vi "WPI_DigitalModuleERRDIOAlreadyAllocated.vi"(8 "error in (no error)":errorcluster, 10 "DIOChannel":T1) -> (0 "error out":errorcluster)   [LabVIEW 2017]
doc: "This software is licensed. Open the labview\\readme\\WPI Robotics Library Open Source License.txt file for more information."
uses:
  <vilib>/Rock Robotics/SystemInterfaces/DIO/FPGA_DIOChannel.ctl
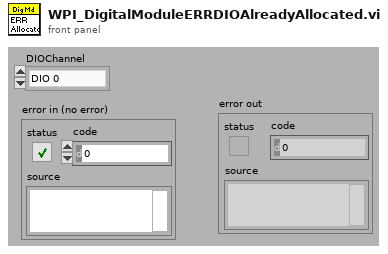
[diagram p1: front panel]
types:
  T1 = typedef "FPGA_DIOChannel.ctl" = enum8{"DIO 0", "DIO 1", "DIO 2", "DIO 3", "DIO 4", "DIO 5", "DIO 6", "DIO 7", "DIO 8", "DIO 9", "DIO MXP 0", "DIO MXP 1", "DIO MXP 2", "DIO MXP 3", "DIO MXP 4", "DIO MXP 5", "DIO MXP 6", "DIO MXP 7", "DIO MXP 8", "DIO MXP 9", "DIO MXP 10", "DIO MXP 11", "DIO MXP 12", "DIO MXP 13", "DIO MXP 14", "DIO MXP 15", "SPI Port CS1", "SPI Port CS2", "SPI Port CS3", "SPI Port MISO", "SPI Port MOSI", "Invalid"}
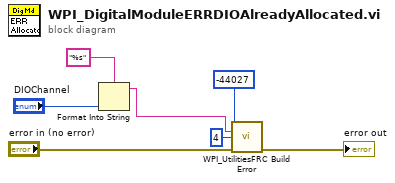
[diagram p0: block diagram]
diagram:
  n1 = Format Into String(format string="%s", "DIOChannel") -> (resulting string=w2:string)  [unwired: 2 in, 1 out]
  n2 = call <vilib>:"WPI_UtilitiesFRC Build Error.vi"("error code"=-44027 ("code"), "extra error text"=w2, "chain levels to remove (1)"=4, "error in (no error)"="error in (no error)") -> ("error out"=→"error out":errorcluster)  [unwired: 1 in, 10 out]
